vi "Ex_Station_Meteo.vi"() -> ()   [LabVIEW 2018]
uses:
  <vilib>/Instr/_visa.llb/VISA Configure Serial Port (Instr).vi
  <vilib>/Utility/file.llb/Write Delimited Spreadsheet (string).vi
panel:
  in  "Chemin De Fichier":path
  in  "Save":bool
  in  "Pause/Play":bool
  out "Waveform Graph 3":dbl[](graph)
  out "Array 3":dbl[](array[numeric])
  out "Waveform Graph 2":dbl[](graph)
  out "Array 2":dbl[](array[numeric])
  out "Waveform Graph":dbl[](graph)
  out "Array":dbl[](array[numeric])
  out "Chaîne":string
  in  "Stop":bool
  in  "Nom de ressource VISA":refnum<visa-resource-name>
  # "1. Brancher la carte Arduino sur un port USB\n2. Choisir le port COM de la carte dans la liste déroulante \"Nom de ressource VISA\"\n3. Lancer le programme"
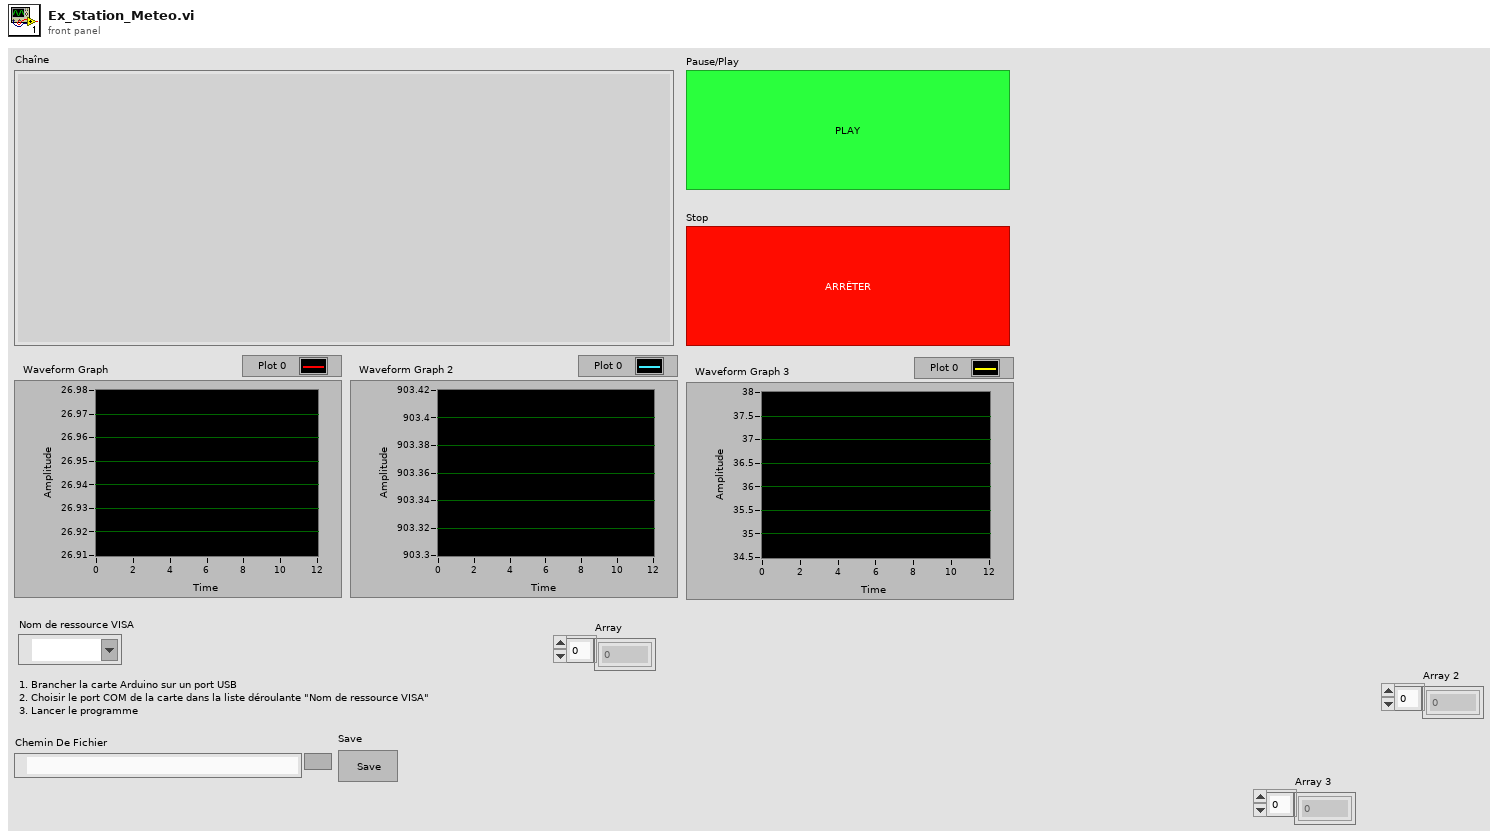
[diagram p1: front panel]
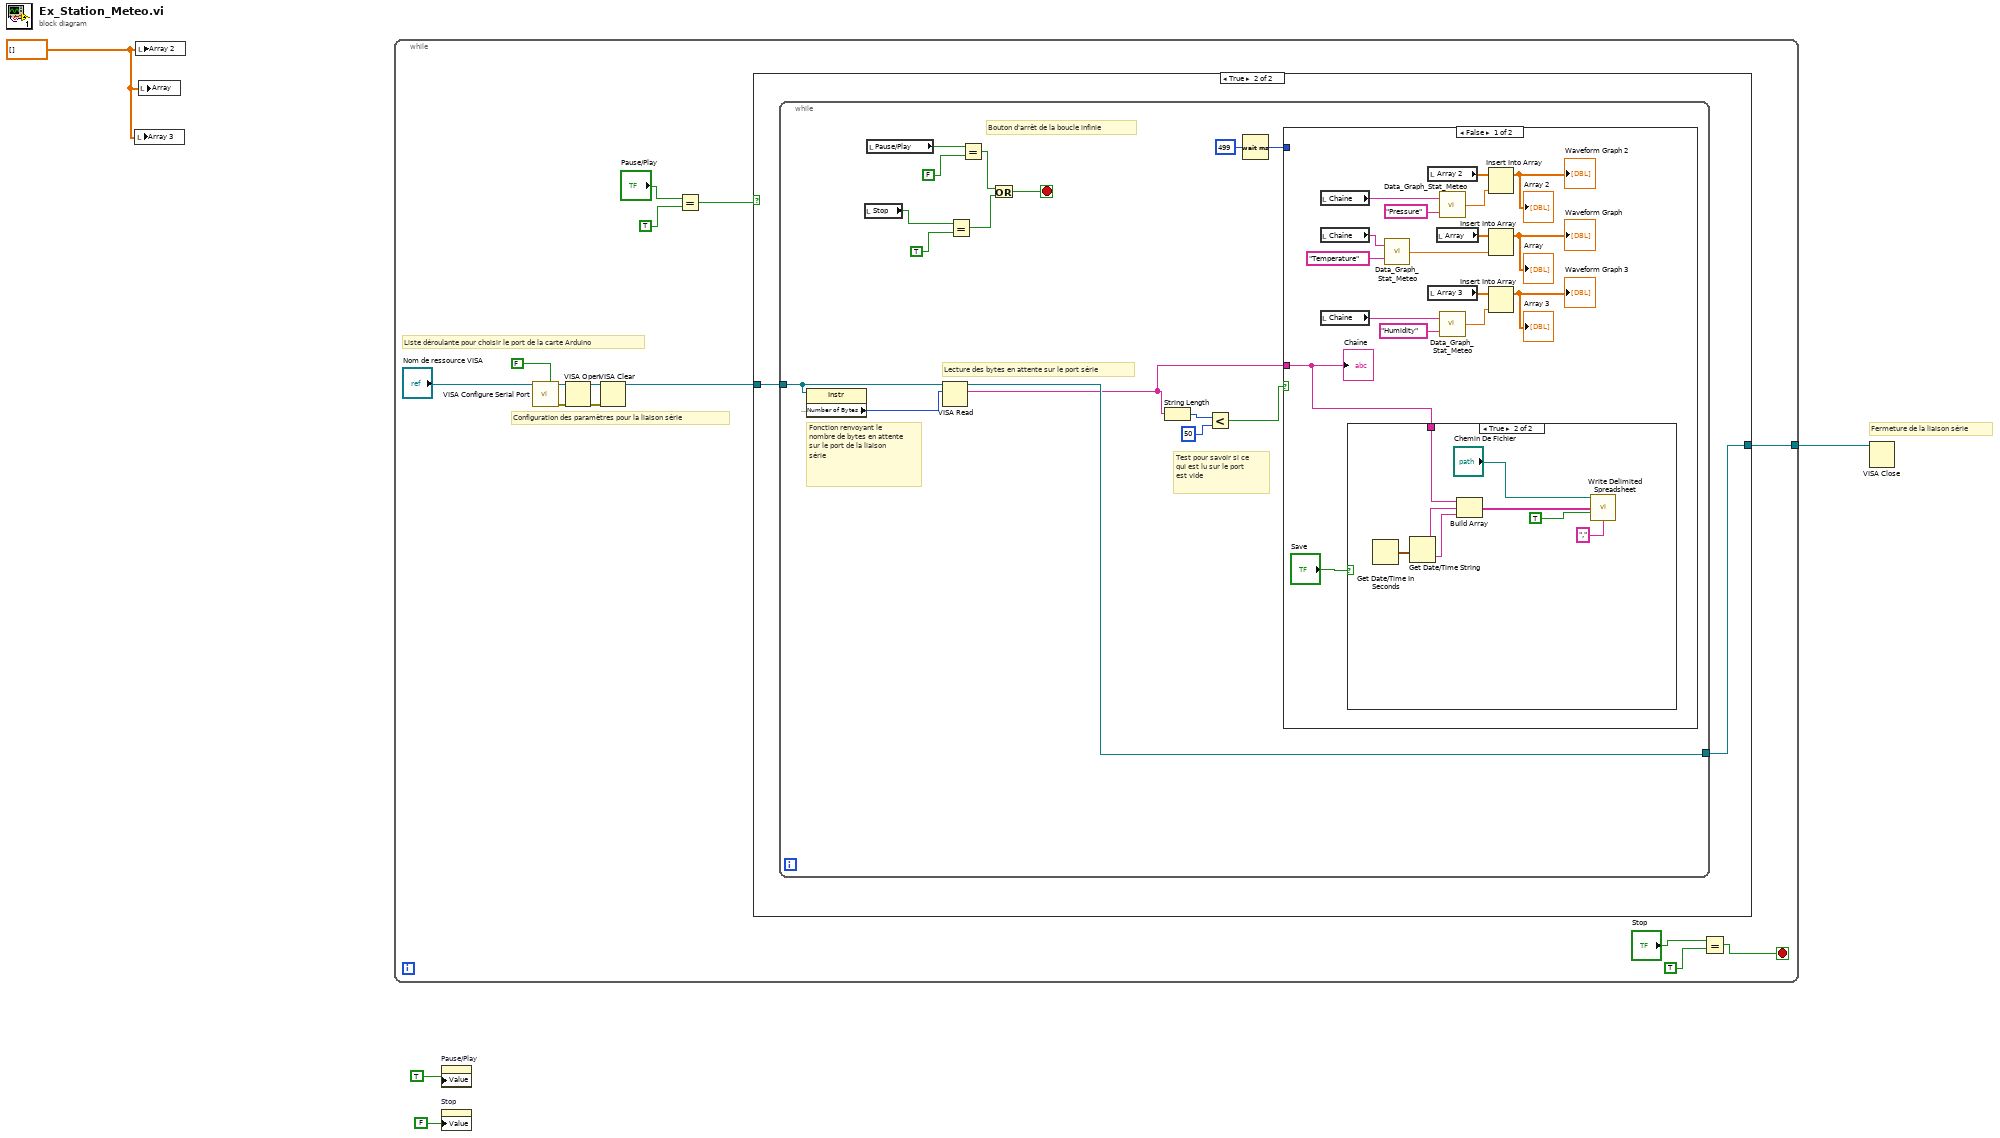
[diagram p0: block diagram]
diagram:
  w3 = dbl[] []
  # "Fermeture de la liaison série"
  n1 = local write "Array 3"(w3) -> ()
  n2 = local write "Array 2"(w3) -> ()
  n3 = local write "Array"(w3) -> ()
  n4 = while {
    tunnel: [w11] -> w4
    stop <- w5 stop-if-true
    # "Configuration des paramètres pour la liaison série"
    # "Liste déroulante pour choisir le port de la carte Arduino"
    n5 = call-poly "VISA Configure Serial Port"("VISA resource name"="Nom de ressource VISA", "Enable Termination\nChar (T)"=FALSE ("Enable Termination\nChar (T)")) -> ("VISA resource name out"=w15:refnum<visa-resource-name>, "error out"=w13:errorcluster)  [unwired: 12 in]
    n6 = VISA Open(error in (no error)=w13, VISA resource name=w15) -> (VISA resource name=w17:refnum<visa-resource-name>, error out=w12:errorcluster)  [unwired: 3 in]
    n7 = VISA Clear(VISA resource name=w17, error in (no error)=w12) -> (VISA resource name out=w16:refnum<visa-resource-name>)  [unwired: 1 out]
    n8 = Equal?(x="Pause/Play", y=TRUE ("Boolean")) -> (x = y?=w8:bool)
    n9 = case shown="True" w8 {
      tunnel: w16 -> [w19 w21]
      tunnel: [w19 w20] -> w11
      frame False {
      }
      frame True {
        n10 = while {
          tunnel: w21 -> [w37]
          tunnel: [w35] -> w20
          stop <- w23 stop-if-true
          # "Lecture des bytes en attente sur le port série"
          # "Fonction renvoyant le nombre de bytes en attente\nsur le port de la liaison série"
          # "Test pour savoir si ce qui est lu sur le port est vide"
          # "Bouton d'arrêt de la boucle infinie"
          n11 = property class="Instr"(reference=w37) -> ("Serial Settings:Number of Bytes at Serial Port"=w36:u32)  [unwired: 1 in, 2 out]
          n12 = local read "Stop"() -> (w26:bool)
          n13 = local read "Pause/Play"() -> (w27:bool)
          n14 = VISA Read(VISA resource name=w37, byte count=w36) -> (VISA resource name out=w35:refnum<visa-resource-name>, read buffer=w32:string)  [unwired: 1 in, 2 out]
          n15 = Equal?(x=w26, y=TRUE ("Boolean")) -> (x = y?=w22:bool)
          n16 = Equal?(x=w27, y=FALSE ("Boolean")) -> (x = y?=w24:bool)
          n17 = Or(x=w24, y=w22) -> (x .or. y?=w23:bool)
          n18 = String Length(string=w32) -> (length=w31:i32)
          n19 = Less?(x=w31, y=50) -> (x < y?=w29:bool)
          n20 = Wait (ms)(milliseconds to wait=u32 499) -> (millisecond timer value=w34:u32)
          n21 = case shown="False" w29 {
            tunnel: w32 -> [w38 _]
            tunnel: w34 -> [_ _]
            frame False {
              n22 = local read "Chaîne"() -> (w46:string)
              n23 = local read "Chaîne"() -> (w54:string)
              n24 = local read "Chaîne"() -> (w41:string)
              n25 = case shown="True" "Save" {
                tunnel: w38 -> [_ w57]
                frame False {
                }
                frame True {
                  n26 = Get Date/Time In Seconds() -> (seconds since 1Jan1904=w62:timestamp)
                  n27 = Get Date/Time String(seconds (now)=w62) -> (date string=w58:string, time string=w59:string)  [unwired: 2 in]
                  n28 = Build Array(w57, w58, w59) -> (w60:string[])
                  n29 = call-poly <vilib>:"Write Delimited Spreadsheet.vi"("file path (dialog if empty)"="Chemin De Fichier", "1D data"=w60, "append to file? (new file:F)"=TRUE, "delimiter (\\t)"="," ("delimiter (\\t)")) -> ()  [unwired: 10 in, 2 out]
                }
              }
              n30 = call "Data_Graph_Stat_Meteo.vi"("mesure cherchée"="Temperature", "Chaine Arduino"=w54) -> ("Numeric"=w52:dbl)
              n31 = local read "Array 2"() -> (w48:dbl[])
              n32 = local read "Array 3"() -> (w43:dbl[])
              n33 = local read "Array"() -> (w51:dbl[])
              n34 = call "Data_Graph_Stat_Meteo.vi"("mesure cherchée"="Pressure", "Chaine Arduino"=w46) -> ("Numeric"=w49:dbl)
              n35 = call "Data_Graph_Stat_Meteo.vi"("mesure cherchée"="Humidity", "Chaine Arduino"=w41) -> ("Numeric"=w44:dbl)
              n36 = Insert Into Array(array=w48, new element=w49) -> (→"Array 2" →"Waveform Graph 2":dbl[])  [unwired: 1 in]
              n37 = Insert Into Array(array=w51, new element=w52) -> (→"Array" →"Waveform Graph":dbl[])  [unwired: 1 in]
              n38 = Insert Into Array(array=w43, new element=w44) -> (→"Array 3" →"Waveform Graph 3":dbl[])  [unwired: 1 in]
              "Chaîne" <- w38
            }
            frame True {
            }
          }
        }
      }
    }
    n39 = Equal?(x="Stop", y=TRUE ("Boolean")) -> (x = y?=w5:bool)
  }
  n40 = property on="Pause/Play" class="Bool (strict)"("Value"=TRUE) -> ()  [unwired: 2 in, 2 out]
  n41 = property on="Stop" class="Bool (strict)"("Value"=FALSE) -> ()  [unwired: 2 in, 2 out]
  n42 = VISA Close(VISA resource name=w4) -> ()  [unwired: 1 in, 1 out]
